vi "Tray_TrayDataToUIByNumber.vi"(0 "TrayInRefIn":refnum<vi>, 1 "ItemFrom":string[](array[string]), 5 "Index":i32, 7 "TrayType":T1, 9 "TraySize":cluster{"y":u32, "x":u32}={"y"=16, "x"=6}, 11 "error in":errorcluster) -> (15 "error out":errorcluster)   [LabVIEW 2015]
uses:
  Tray_TrayName.ctl
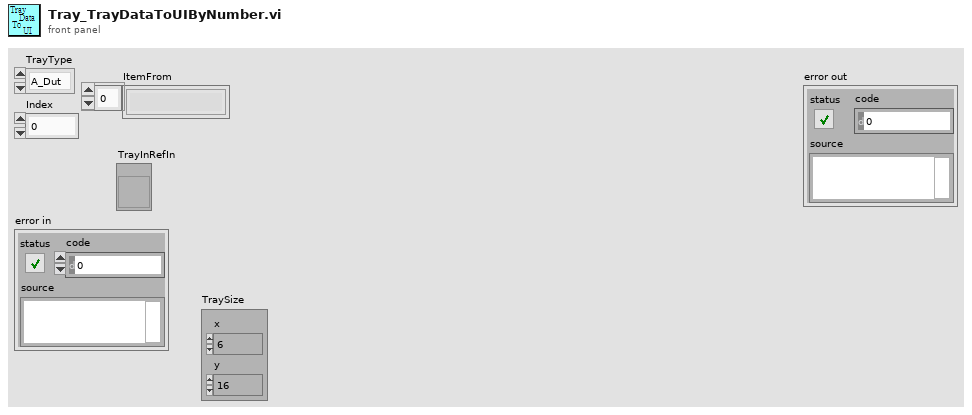
[diagram p1: front panel]
types:
  T1 = typedef "Tray_TrayName.ctl" = enum16{"A_Dut", "B_Pass", "C_NGR", "D_NGL"}
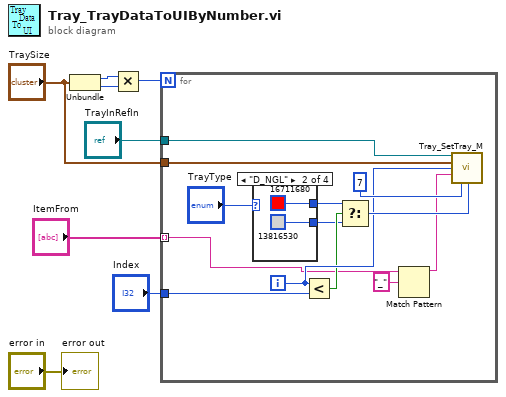
[diagram p0: block diagram]
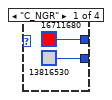
[diagram p2: hidden frame]
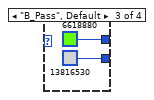
[diagram p3: hidden frame]
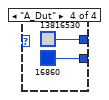
[diagram p4: hidden frame]
diagram:
  n1 = Unbundle("TraySize") -> ("y"=w3:u32, "x"=w4:u32)
  n2 = Multiply(x=w3, y=w4) -> (x*y=w2:u32)
  n3 = for {
    N: w2 -> [_]
    tunnel: "TrayInRefIn" -> [w18]
    tunnel: "TraySize" -> [w17]
    tunnel: "Index" -> [w14]
    tunnel: "ItemFrom" -> [w11] mode=indexing
    i -> [w15]
    n4 = case shown="\"D_NGL\"" "TrayType" {
      tunnel: [u32 16711680 ("Initial color") u32 16711680 ("Initial color") u32 6618880 ("Initial color") u32 13816530 ("Initial color")] -> w20
      tunnel: [u32 13816530 ("Initial color") u32 13816530 ("Initial color") u32 13816530 ("Initial color") u32 16860 ("Initial color")] -> w12
      frame "C_NGR" {
      }
      frame "D_NGL" {
      }
      frame "B_Pass", Default {
      }
      frame "A_Dut" {
      }
    }
    n5 = Less?(x=w15, y=w14) -> (x < y?=w13:bool)
    n6 = Select(t=w20, s=w13, f=w12) -> (s? t:f=w19:u32)
    n7 = Match Pattern(string=w11, regular expression="_") -> (before substring=w10:string)  [unwired: 1 in, 3 out]
    n8 = call "Tray_SetTray_M.vi"("TrayIn"=w18, "GridSize"=w17, "Index Number"=w15, "String"=w10, "Direction"=u16 7, "Color Box"=w19) -> ()  [unwired: 9 in, 1 out]
  }
  "error out" <- "error in"
